vi "receive.vi"(8 "error in (no error)":errorcluster, 11 "IModbus in":refnum<class "IModbus.lvclass">) -> (0 "error out":errorcluster, 2 "Data":T1[](array[typedef]) {"Data" format="%02x"}, 3 "IModbus out":refnum<class "IModbus.lvclass">)   [LabVIEW 2016, in "RTModbus.lvlib" / "IModbus.lvclass"]
uses:
  IModbus.lvclass
  DataTypes/RxFrame.ctl
  RTModbus.lvlib
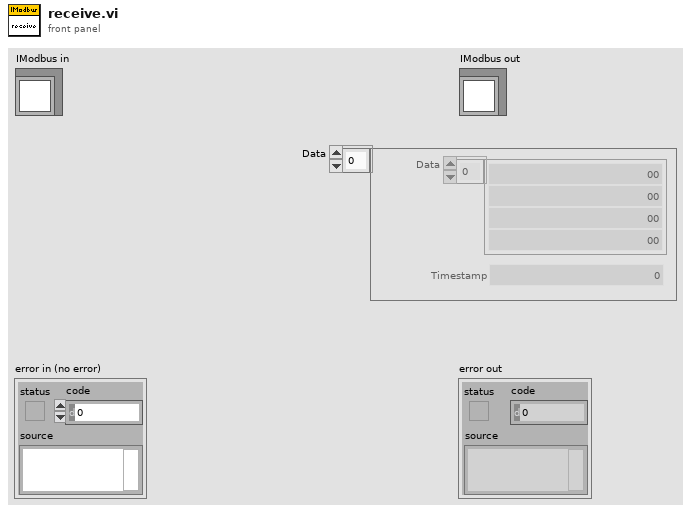
[diagram p1: front panel]
types:
  T1 = typedef "RTModbus.lvlib/RxFrame.ctl" = cluster{"Data":u8[], "Timestamp":u64}
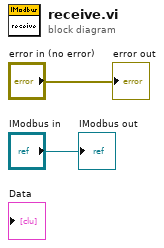
[diagram p0: block diagram]
diagram:
  "error out" <- "error in (no error)"
  "IModbus out" <- "IModbus in"
